vi "R1CleanUp.vi"(8 "error in (no error)":errorcluster) -> (0 "error out":errorcluster)   [LabVIEW 2016]
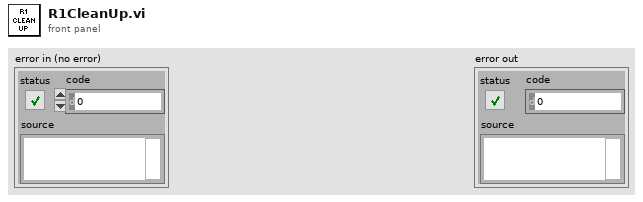
[diagram p1: front panel]
types:
  T1 = cluster{"Media Pump":bool, "Water Pump":bool, "Gas Pump":bool, "Effluent Pump":bool}
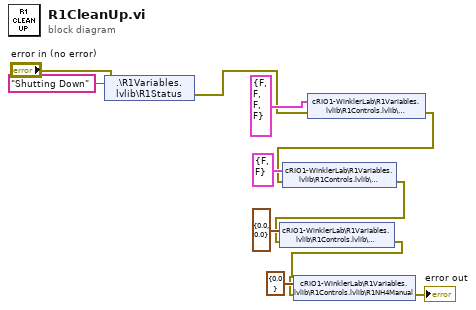
[diagram p0: block diagram]
diagram:
  n1 = shared-variable ".\\R1Variables.lvlib\\R1Status"("Shutting Down" ("R1Status"), error in="error in (no error)") -> (error out=w6:errorcluster)
  n2 = shared-variable "cRIO1-WinklerLab\\R1Variables.lvlib\\R1Controls.lvlib\\R1SBRManual"(T1 {"Media Pump"=FALSE, "Water Pump"=FALSE, "Gas Pump"=FALSE, "Effluent Pump"=FALSE} ("R1SBR_Manual"), error in=w6) -> (error out=w3:errorcluster)
  n3 = shared-variable "cRIO1-WinklerLab\\R1Variables.lvlib\\R1Controls.lvlib\\R1pHManual"(cluster{"Acid Pump":bool, "Base Pump":bool} {"Acid Pump"=FALSE, "Base Pump"=FALSE} ("R1pHManual"), error in=w3) -> (error out=w2:errorcluster)
  n4 = shared-variable "cRIO1-WinklerLab\\R1Variables.lvlib\\R1Controls.lvlib\\R1DOManual"(cluster{"Air MFC":dbl, "N2 MFC":dbl} {"Air MFC"=0.0, "N2 MFC"=0.0} ("R1DOManual"), error in=w2) -> (error out=w1:errorcluster)
  n5 = shared-variable "cRIO1-WinklerLab\\R1Variables.lvlib\\R1Controls.lvlib\\R1NH4Manual"(cluster{"NH4 Pump Flowrate, ml/min":dbl} {"NH4 Pump Flowrate, ml/min"=0.0} ("R1NH4Manual"), error in=w1) -> (error out=→"error out":errorcluster)
